vi "Tote_Sensor_Detect.vi"(8 "Tote_Detect_2":T1, 9 "Tote_Detect_1":T1) -> (2 "Tote_Detect_2":bool, 3 "Tote_Detect_1":bool)   [LabVIEW 2014]
uses:
  <vilib>/Rock Robotics/WPI/AnalogChannel/WPI_AnalogChannelDevRef.ctl
  <vilib>/Rock Robotics/SystemInterfaces/Typedef/FPGA_TypedefAnalogModule.ctl
  <vilib>/Rock Robotics/SystemInterfaces/AI/FPGA_AIChannel.ctl
panel:
  out "?":cluster{dbl, dbl}(graph)
  in  "Detect_Tote_Thresh_Hold":dbl=1.0
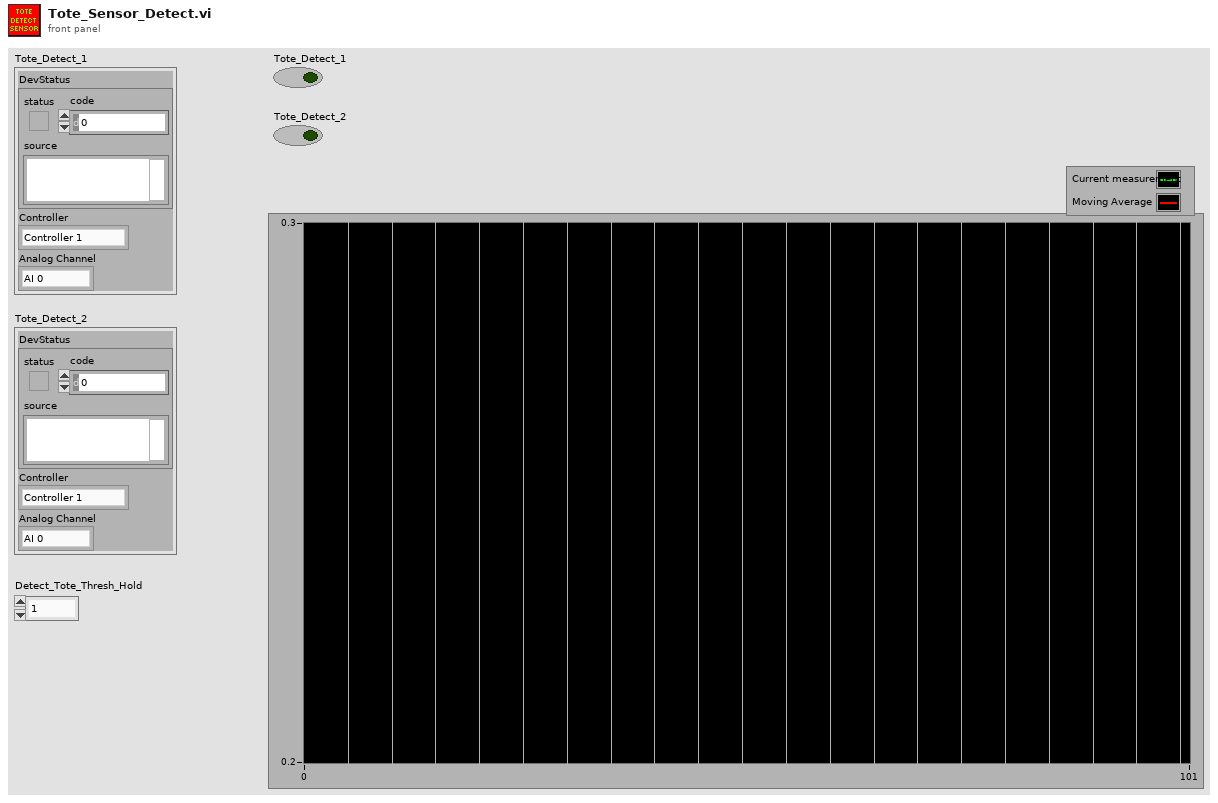
[diagram p1: front panel]
types:
  T1 = typedef "WPI_AnalogChannelDevRef.ctl" = cluster{"DevStatus":errorcluster, "Controller":T2, "Analog Channel":T3}
  T2 = typedef "FPGA_TypedefAnalogModule.ctl" = enum16{"Controller 1"}
  T3 = typedef "FPGA_AIChannel.ctl" = enum8{"AI 0", "AI 1", "AI 2", "AI 3", "AI MXP 0", "AI MXP 1", "AI MXP 2", "AI MXP 3", "Invalid"}
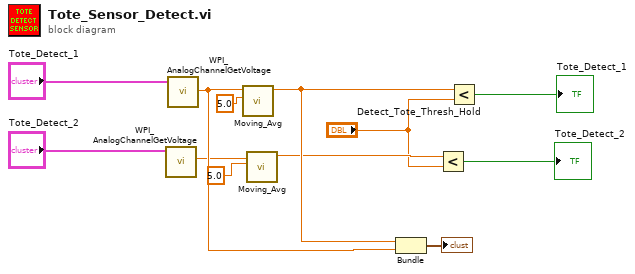
[diagram p0: block diagram]
diagram:
  n1 = call <vilib>:"WPI_AnalogChannelGetVoltage.vi"("AIDeviceRef"="Tote_Detect_2") -> ("Voltage"=w7:dbl)  [unwired: 8 in, 2 out]
  n2 = call <vilib>:"WPI_AnalogChannelGetVoltage.vi"("AIDeviceRef"="Tote_Detect_1") -> ("Voltage"=w12:dbl)  [unwired: 8 in, 2 out]
  n3 = call "Moving_Avg.vi"("Num_Avg"=5.0, "Numeric in"=w12) -> ("Numeric out"=w11:dbl)  [unwired: 9 in]
  n4 = call "Moving_Avg.vi"("Num_Avg"=5.0, "Numeric in"=w7) -> ("Numeric out"=w9:dbl)  [unwired: 9 in]
  n5 = Bundle("Numeric out"=w11, "Voltage"=w12) -> (→"?":cluster{"Numeric out":dbl, "Voltage":dbl})  [unwired: 1 in]
  n6 = Less?(x=w9, y="Detect_Tote_Thresh_Hold") -> (x < y?=→"Tote_Detect_2":bool)
  n7 = Less?(x=w11, y="Detect_Tote_Thresh_Hold") -> (x < y?=→"Tote_Detect_1":bool)
